vi "aim white.vi"(8 "error in (no error)":errorcluster, 11 "KNR in":T2) -> (0 "error out":errorcluster, 3 "KNR out":T2, 4 "DC Position Offset":i32)   [LabVIEW 2013]
uses:
  <userlib>/KNR OS 3.0 LabVIEW Toolkit/Type Definition/KNR3 Reference.ctl
  <userlib>/_FPGA Interface Advanced Tools/FPGA Interface Base/FPGA Interface Base.lvclass
  <userlib>/KNR OS 3.0 LabVIEW Toolkit/Type Definition/Resource.ctl
  Global 1.vi
panel:
  out "处理前":T1(plugin-control)
  out "中心坐标与对应的面积":dbl[][](array[numeric])
  out "处理后":T1(plugin-control)
  out "Error(deg)":ext
  in  "STOP":bool
  out "CM":dbl
  out "e pix":dbl
  out "Aim":dbl
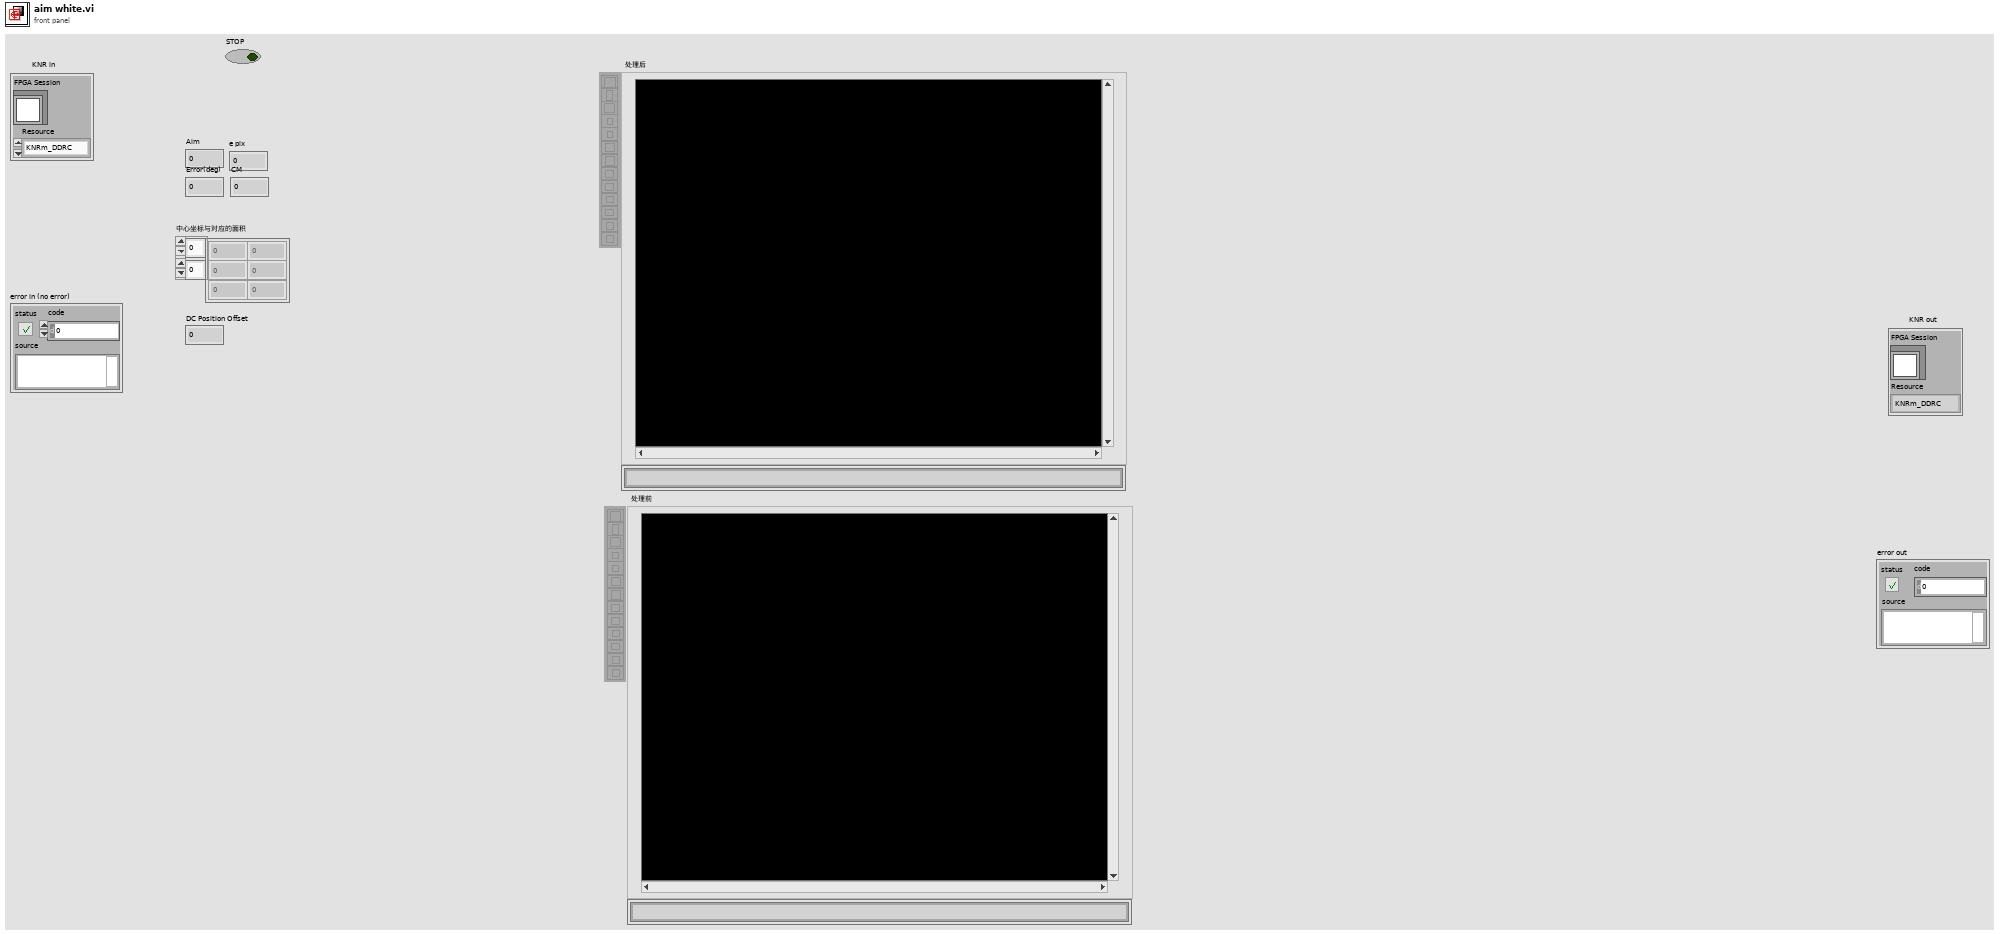
[diagram p1: front panel]
types:
  T1 = typedef "IMAQ Image.ctl" = refnum<image>
  T2 = typedef "KNR3 Reference.ctl" = cluster{"FPGA Session":refnum<class "FPGA Interface Base.lvclass">, "Resource":T3}
  T3 = typedef "Resource.ctl" = enum16{"KNRm_DDRC", "KNRm_DDDD", "KNRm_DDDR", "KNRm_DDDC", "KNR"}
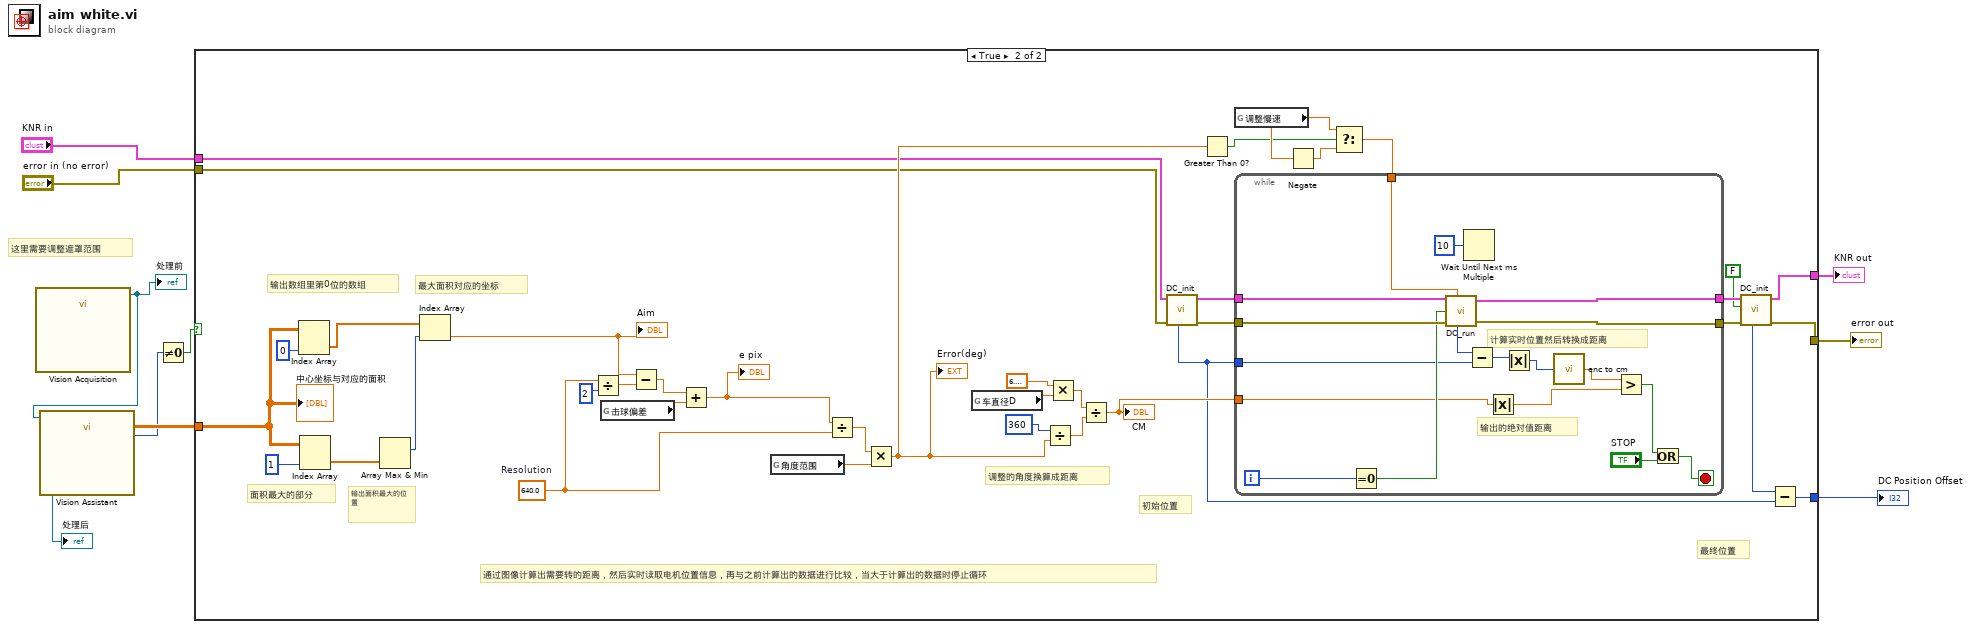
[diagram p0: block diagram]
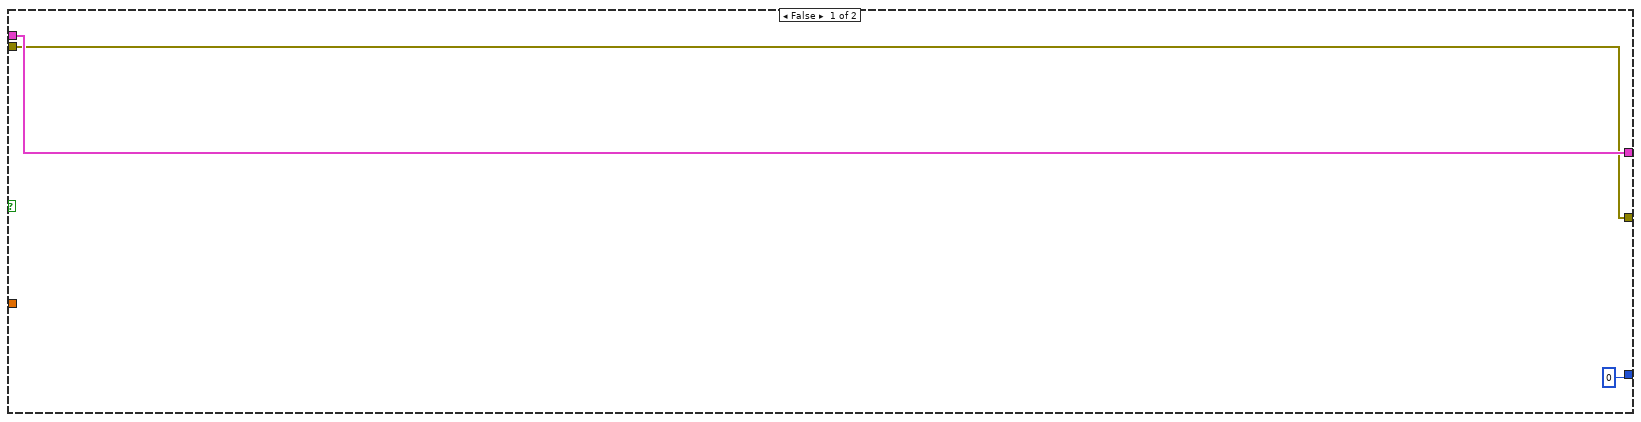
[diagram p2: hidden frame]
diagram:
  # "这里需要调整遮罩范围"
  n1 = call "Vision Acquisition"() -> ("Image Out"=w1:T1)  [unwired: 26 in, 1 out]
  "处理前" <- w1
  n2 = call "Vision Assistant"("Image In"=w1) -> ("Image Out"=→"处理后":T1, "Particle Measurements (Pixels) (Particle Analysis 1)"=w7:dbl[][], "Number of Particles (Particle Analysis 1)"=w4:i32)  [unwired: 23 in, 1 out]
  n3 = Not Equal To 0?(x=w4) -> (x != 0?=w5:bool)
  n4 = case shown="True" w5 {
    tunnel: [w13 w25] -> w10
    tunnel: [w12 w24] -> w9
    tunnel: w7 -> [_ w18]
    tunnel: [0 w16] -> w6
    tunnel: "KNR in" -> [w13 w15]
    tunnel: "error in (no error)" -> [w12 w14]
    frame False {
    }
    frame True {
      w35 = 640.0  # Resolution
      # "最终位置"
      # "最大面积对应的坐标"
      # "面积最大的部分"
      # "输出面积最大的位置"
      # "输出数组里第0位的数组"
      # "调整的角度换算成距离"
      # "初始位置"
      # "通过图像计算出需要转的距离，然后实时读取电机位置信息，再与之前计算出的数据进行比较，当大于计算出的数据时停止循环"
      n5 = Index Array(array=w18, index (col)=0 ("disabled index (col)")) -> (element=w21:dbl[])  [unwired: 1 in]
      n6 = Index Array(array=w18, index (col)=1 ("disabled index (col)")) -> (element=w20:dbl[])  [unwired: 1 in]
      n7 = Array Max & Min(array=w20) -> (max index (indices)=w19:i32)  [unwired: 3 out]
      n8 = Index Array(array=w21, index=w19) -> (element=w17:dbl)
      "Aim" <- w17
      n9 = Divide(x=w35, y=2) -> (x/y=w34:dbl)
      n10 = global read "Global 1.vi" "击球偏差"() -> (w50:dbl)
      n11 = Subtract(x=w17, y=w34) -> (x-y=w51:dbl)
      n12 = Add(x=w51, y=w50) -> (x+y=w47:dbl)
      "e pix" <- w47
      n13 = global read "Global 1.vi" "角度范围"() -> (w49:dbl)
      n14 = Divide(x=w47, y=w35) -> (x/y=w48:dbl)
      n15 = Multiply(x=w48, y=w49) -> (x*y=w28:dbl)
      "Error(deg)" <- w28
      n16 = global read "Global 1.vi" "车直径D"() -> (w44:dbl)
      n17 = Divide(x=360, y=w28) -> (x/y=w42:dbl)
      n18 = Multiply(x=6.283185307179586, y=w44) -> (x*y=w43:dbl)
      n19 = Divide(x=w43, y=w42) -> (x/y=w39:dbl)
      "CM" <- w39
      n20 = call "DC_init.vi"("error in (no error)"=w14, "KNR in"=w15) -> ("error out"=w40:errorcluster, "KNR out"=w41:T2, "output\nPosition_1"=w32:i32)  [unwired: 6 in, 1 out]
      n21 = Greater Than 0?(x=w28) -> (x > 0?=w29:bool)
      n22 = global read "Global 1.vi" "调整慢速"() -> (w30:dbl)
      n23 = Negate(x=w30) -> (-x=w31:dbl)
      n24 = Select(t=w30, s=w29, f=w31) -> (s? t:f=w27:dbl)
      n25 = while {
        tunnel: w41 -> [w69]
        tunnel: w40 -> [w68]
        tunnel: [w67] -> w38
        tunnel: [w66] -> w37
        tunnel: w39 -> [w57]
        tunnel: w32 -> [w54]
        tunnel: w27 -> [w52]
        i -> [w60]
        stop <- w63 stop-if-true
        # "输出的绝对值距离"
        # "计算实时位置然后转换成距离"
        n26 = Equal To 0?(x=w60) -> (x = 0?=w59:bool)
        n27 = call "DC_run.vi"("KNR in"=w69, "speed_1"=w52, "reinitialize? (F)"=w59, "error in (no error)"=w68) -> ("Position_1"=w53:i32, "KNR out"=w67:T2, "error out"=w66:errorcluster)  [unwired: 2 in, 1 out]
        n28 = Wait Until Next ms Multiple(millisecond multiple=u32 10) -> ()  [unwired: 1 out]
        n29 = Subtract(x=w53, y=w54) -> (x-y=w65:i32)
        n30 = Absolute Value(x=w57) -> (abs(x)=w64:dbl)
        n31 = Absolute Value(x=w65) -> (abs(x)=w56:i32)
        n32 = call "enc to cm.vi"("E"=w56) -> ("CM"=w55:dbl)  [unwired: 1 in]
        n33 = Greater?(x=w55, y=w64) -> (0:w62:bool)
        n34 = Or(x=w62, y="STOP") -> (x .or. y?=w63:bool)
      }
      n35 = call "DC_init.vi"("error in (no error)"=w37, "Enable Motor(T)"=FALSE, "KNR in"=w38) -> ("error out"=w24:errorcluster, "KNR out"=w25:T2, "output\nPosition_1"=w26:i32)  [unwired: 5 in, 1 out]
      n36 = Subtract(x=w26, y=w32) -> (x-y=w16:i32)
      "中心坐标与对应的面积" <- w18
    }
  }
  "error out" <- w9
  "KNR out" <- w10
  "DC Position Offset" <- w6
